vi "ConfigInstr.vi"(6 "InstrumentName":string, 7 "VisaRessIn":refnum<visa-resource-name>="GPIB0::12::INSTR", 8 "error in (no error)":errorcluster caption="entrée d'erreur (pas d'erreur)", 9 "FirstClassInst":bool, 10 "Function":string, 11 "EG_G5210 In":refnum<class "EGG5210.lvclass"> caption="DNL_LabVIEW Object in") -> (0 "error out":errorcluster caption="sortie d'erreur", 3 "EG_G5210 Out":refnum<class "EGG5210.lvclass"> caption="DNL_LabVIEW Object out")   [LabVIEW 2019, in "EGG5210.lvclass"]
uses:
  EGG5210.lvclass
  C:/Programmes Labview/LabScanV1A/DevicesClass/BaseDevice/BaseDevice.lvclass
  EGG5210_Func.ctl
  EGG5210.lvclass/EGG5210.ctl
  BaseDevice/BaseDevice.lvclass/BaseDevice.ctl
  BaseDevice/Accessor/SetShowInstrNm.vi
panel:
  in  "EG_G5210_Func":T1
  out "VisaRessOut":refnum<visa-resource-name>
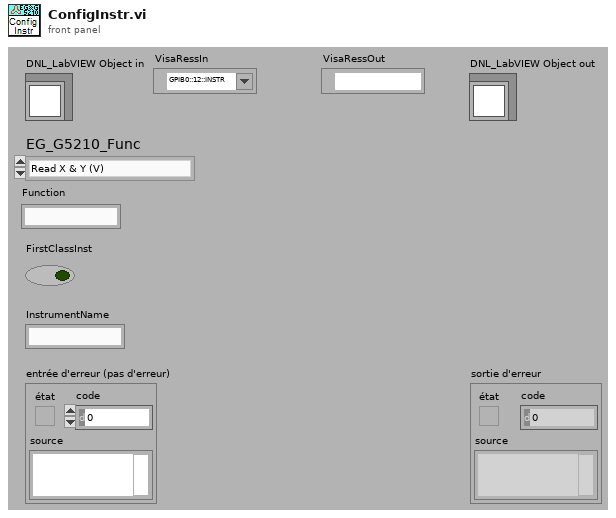
[diagram p1: front panel]
types:
  T1 = typedef "EGG5210.lvclass/EGG5210_Func.ctl" = enum16{"Read X & Y (V)", "Read Mag & Phase (V,°)", "Read X, Y, Mag & Phase (V,V,V,°)", "Read ADC Ch1 (V)", "Read ADC Ch2 (V)", "Oscillator Ctrl (Hz, mV rms)", "PL Excimer Settings (Na)"}
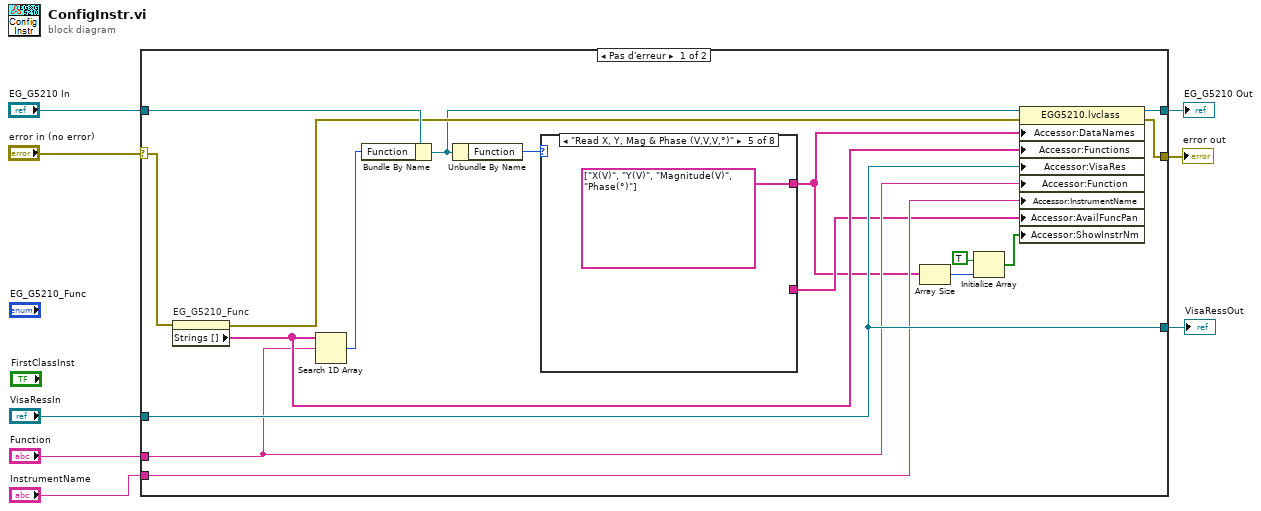
[diagram p0: block diagram]
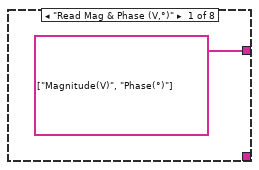
[diagram p2: hidden frame]
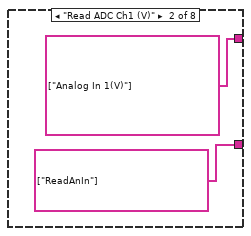
[diagram p3: hidden frame]
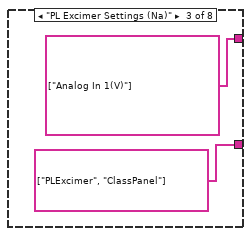
[diagram p4: hidden frame]
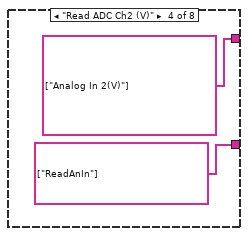
[diagram p5: hidden frame]
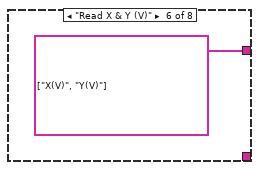
[diagram p6: hidden frame]
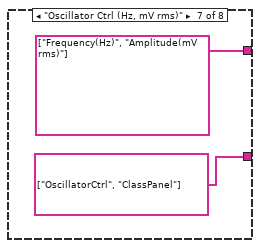
[diagram p7: hidden frame]
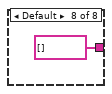
[diagram p8: hidden frame]
diagram:
  n1 = case shown="Pas d'erreur" "error in (no error)" {
    selector: "error in (no error)" -> [w22 w39]
    tunnel: [w20 w39] -> w7
    tunnel: "EG_G5210 In" -> [w24 w38]
    tunnel: [w21 w38] -> w5
    tunnel: "Function" -> [w15 _]
    tunnel: "VisaRessIn" -> [w17 _]
    tunnel: [w17 _] -> w2
    tunnel: "InstrumentName" -> [w14 _]
    frame No Error {
      n2 = property on="EG_G5210_Func" class="Énum (strict)"(error in=w22) -> (error out=w23:errorcluster, "Strings []"=w16:string[])  [unwired: 1 in, 1 out]
      n3 = Search 1D Array(1D array=w16, element=w15) -> (index of element=w25:i32)  [unwired: 1 in]
      n4 = Bundle By Name(cluster=w24, "Function"=w25) -> (w19:refnum<class "EGG5210.lvclass">)
      n5 = Unbundle By Name(w19) -> ("Function"=w18:T1)
      n6 = case shown="\"Read X, Y, Mag & Phase (V,V,V,°)\"" w18 {
        tunnel: [string[] ["Magnitude(V)", "Phase(°)"] string[] ["Analog In 1(V)"] string[] ["Analog In 1(V)"] string[] ["Analog In 2(V)"] string[] ["X(V)", "Y(V)", "Magnitude(V)", "Phase(°)"] string[] ["X(V)", "Y(V)"] string[] ["Frequency(Hz)", "Amplitude(mV rms)"] string[] []] -> w9
        tunnel: [_ string[] ["ReadAnIn"] string[] ["PLExcimer", "ClassPanel"] string[] ["ReadAnIn"] _ _ string[] ["OscillatorCtrl", "ClassPanel"] _] -> w13
        frame "Read Mag & Phase (V,°)" {
        }
        frame "Read ADC Ch1 (V)" {
        }
        frame "PL Excimer Settings (Na)" {
        }
        frame "Read ADC Ch2 (V)" {
        }
        frame "Read X, Y, Mag & Phase (V,V,V,°)" {
        }
        frame "Read X & Y (V)" {
        }
        frame "Oscillator Ctrl (Hz, mV rms)" {
        }
        frame Default {
        }
      }
      n7 = Array Size(array=w9) -> (size(s)=w12:i32)
      n8 = Initialize Array(TRUE, w12) -> (w10:bool[])
      n9 = property class="EGG5210.lvclass"(reference=w19, error in=w23, "Accessor:DataNames"=w9, "Accessor:Functions"=w16, "Accessor:VisaRes"=w17, "Accessor:Function"=w15, "Accessor:InstrumentName"=w14, "Accessor:AvailFuncPan"=w13, "Accessor:ShowInstrNm"=w10) -> (reference out=w21:refnum<class "EGG5210.lvclass">, error out=w20:errorcluster)
    }
    frame Error {
    }
  }
  "error out" <- w7
  "EG_G5210 Out" <- w5
  "VisaRessOut" <- w2
